vi "delay_block.vi"(10 "gain":dbl=1.0, 11 "signal":dbl) -> (3 "signal_out":dbl)   [LabVIEW 2017]
panel:
  in  "Tab Control":enum32{"Page 1", "Page 2"}(tab)
  out "error out":errorcluster
  in  "error in (no error)":errorcluster
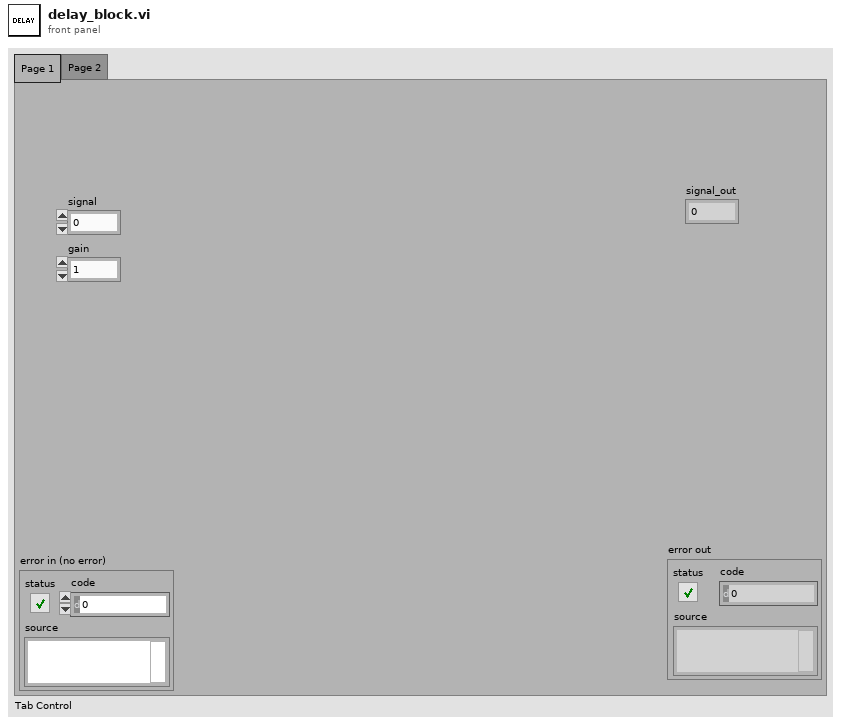
[diagram p1: front panel]
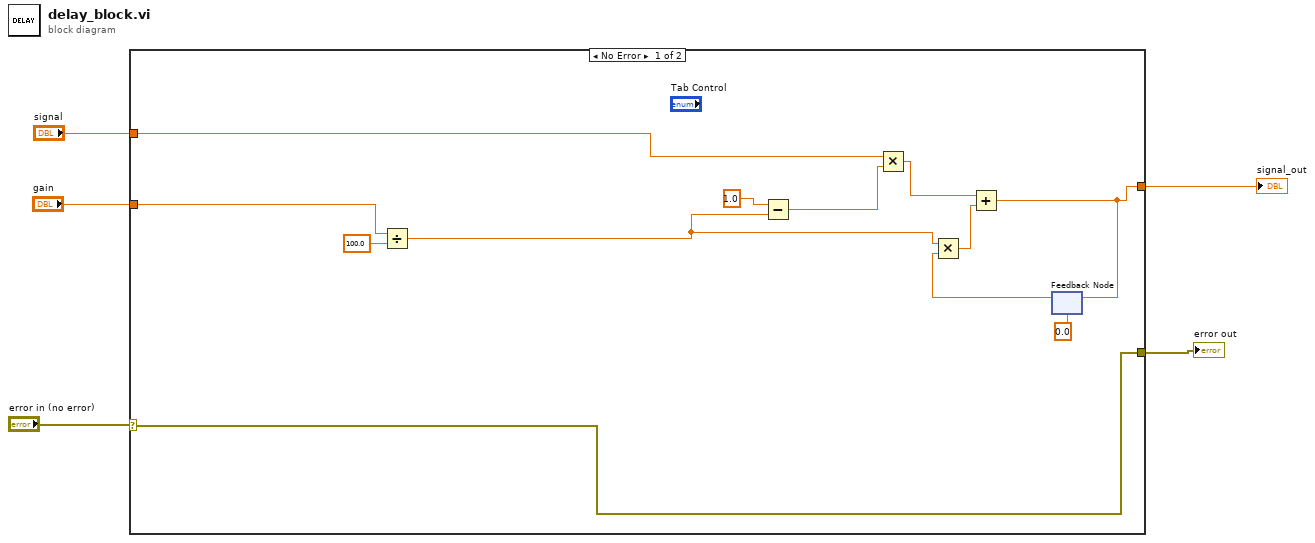
[diagram p0: block diagram]
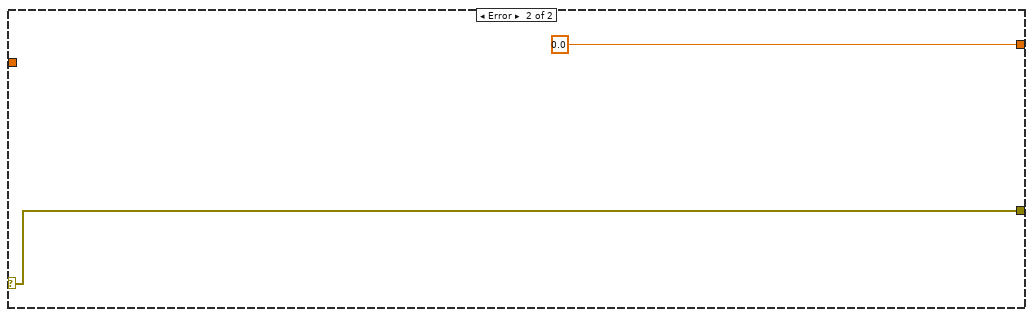
[diagram p2: hidden frame]
diagram:
  n1 = case shown="No Error" "error in (no error)" {
    selector: "error in (no error)" -> [w10 w19]
    tunnel: "signal" -> [w16 _]
    tunnel: "gain" -> [w8 _]
    tunnel: [w14 0.0] -> w3
    tunnel: [w10 w19] -> w1
    frame No Error {
      n2 = Divide(x=w8, y=100.0) -> (x/y=w6:dbl)
      n3 = Subtract(x=1.0, y=w6) -> (x-y=w9:dbl)
      n4 = Multiply(x=w16, y=w9) -> (x*y=w15:dbl)
      n5 = feedback #1(0.0) -> (w13:dbl)
      n6 = Multiply(x=w6, y=w13) -> (x*y=w12:dbl)
      n7 = Add(x=w15, y=w12) -> (x+y=w14:dbl)
      n8 = feedback-in #1(w14) -> ()
    }
    frame Error {
    }
  }
  "signal_out" <- w3
  "error out" <- w1
